vi "cook.vi"(8 "error in (no error)":errorcluster, 11 "Sauté in":refnum<class "Sauté.lvclass">) -> (0 "error out":errorcluster, 3 "Sauté out":refnum<class "Sauté.lvclass">)   [LabVIEW 2010, in "CookBehaviors.lvlib" / "Sauté.lvclass"]
uses:
  Sauté.lvclass
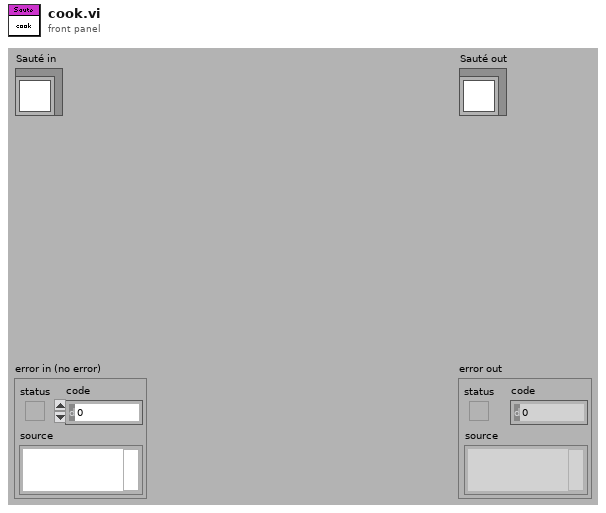
[diagram p1: front panel]
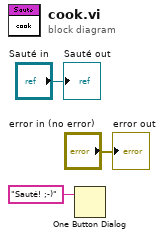
[diagram p0: block diagram]
diagram:
  n1 = One Button Dialog(message="Sauté! ;-)") -> ()  [unwired: 1 in, 1 out]
  "error out" <- "error in (no error)"
  "Sauté out" <- "Sauté in"
